vi "fucking PID.vi"(4 "lorentzian":T1={"Amplitude"=0.011556077084443558, "omega(0)"=1994480.3546612726, "Gamma"=468.65303298958196, "phase"=4.673413347310273, "Q"=4255.771784806969, "Norm  Ampl"=nan, "z (inf)"=2.6527949823343002e-05+0.0007477540585896028i, "4corners"={"z (-pi/2)"=9.277908004825974e-07+0.0007240755403629966i, "z(inf)"=2.6527949823343002e-05+0.0007477540585896028i, "z (pi/2)"=2.8494315967368497e-06+0.0007733542176124632i, "z center"=1.8886111986097237e-06+0.0007487148789877299i, "z(0)"=-2.2750727426123552e-05+0.000749675699385857i, "radius"=2.4658065287076567e-05}} {"z (inf)" format="%#9_9f"; "Q" format="%#9_9f"; "phase" format="%#9_9f"; "Gamma" format="%#9_9f"; "omega(0)" format="%#9_9f"}, 6 "requested size":i32=100, 7 "PID action":T3, 8 "voltage in (V)":cdb=-1.0+0.0i format="%#_10f", 9 "PID parameters":T4={"P (sec)"=-1.0, "I (sec)"=-1.0}, 10 "time in (sec)":dbl=-1.0, 11 "frequency in (Hz)":dbl=-1.0 format="%#_10f") -> (3 "frequency out (Hz)":dbl format="%#_10f")   [LabVIEW 2016]
uses:
  pid -- parameters.ctl
  agregator -- action.ctl
  lorentzian.ctl
  circle corners.ctl
  four-corner circle transformation.ctl
  Q -- check range -- i -- real.vi
  linear interpolation - real.vi
  Q - not nan -- real.vi
panel:
  out "delta theta":dbl
  out "actual number of elements":i32
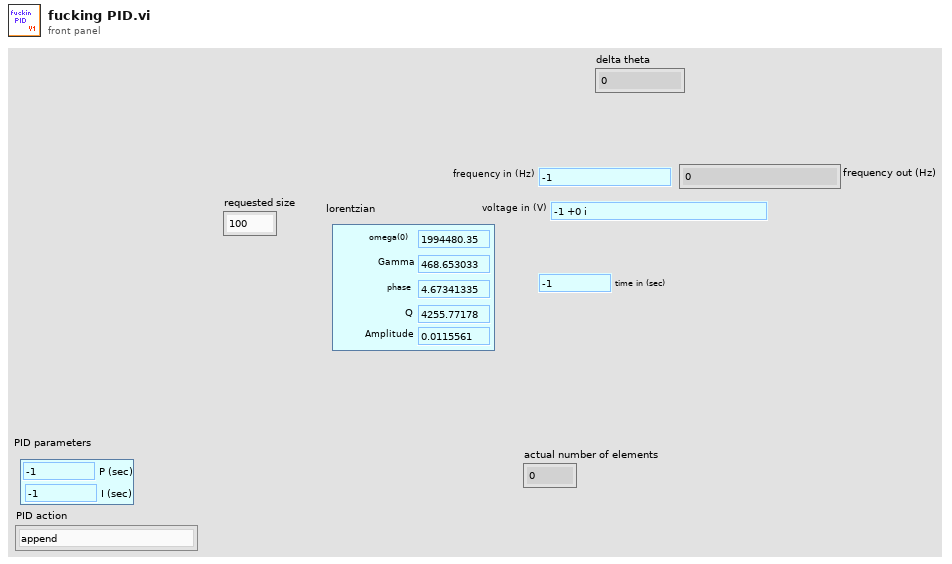
[diagram p1: front panel]
types:
  T1 = typedef "lorentzian.ctl" = cluster{"Amplitude":dbl, "omega(0)":dbl, "Gamma":dbl, "phase":dbl, "Q":dbl, "Norm  Ampl":dbl, "z (inf)":cdb, "4corners":T2}
  T2 = typedef "circle corners.ctl" = cluster{"z (-pi/2)":cdb, "z(inf)":cdb, "z (pi/2)":cdb, "z center":cdb, "z(0)":cdb, "radius":dbl}
  T3 = typedef "agregator -- action.ctl" = enum16{"append", "interpolate", "empty!", "force", "init", "scale", "read last"}
  T4 = typedef "pid -- parameters.ctl" = cluster{"P (sec)":dbl, "I (sec)":dbl}
  T5 = typedef "four-corner circle transformation.ctl" = enum16{"z(c) z(inf)", "z(c) z(zero)", "fix phase", "calculate lorentzian", "z(0) z(+-pi/2)", "shift to zcenter", "to  canonical", "get canonical phase"}
  T6 = typedef "interpolation state - real.ctl" = cluster{"requested size":i32, "Array":dbl[], "actual number of elements":i32}
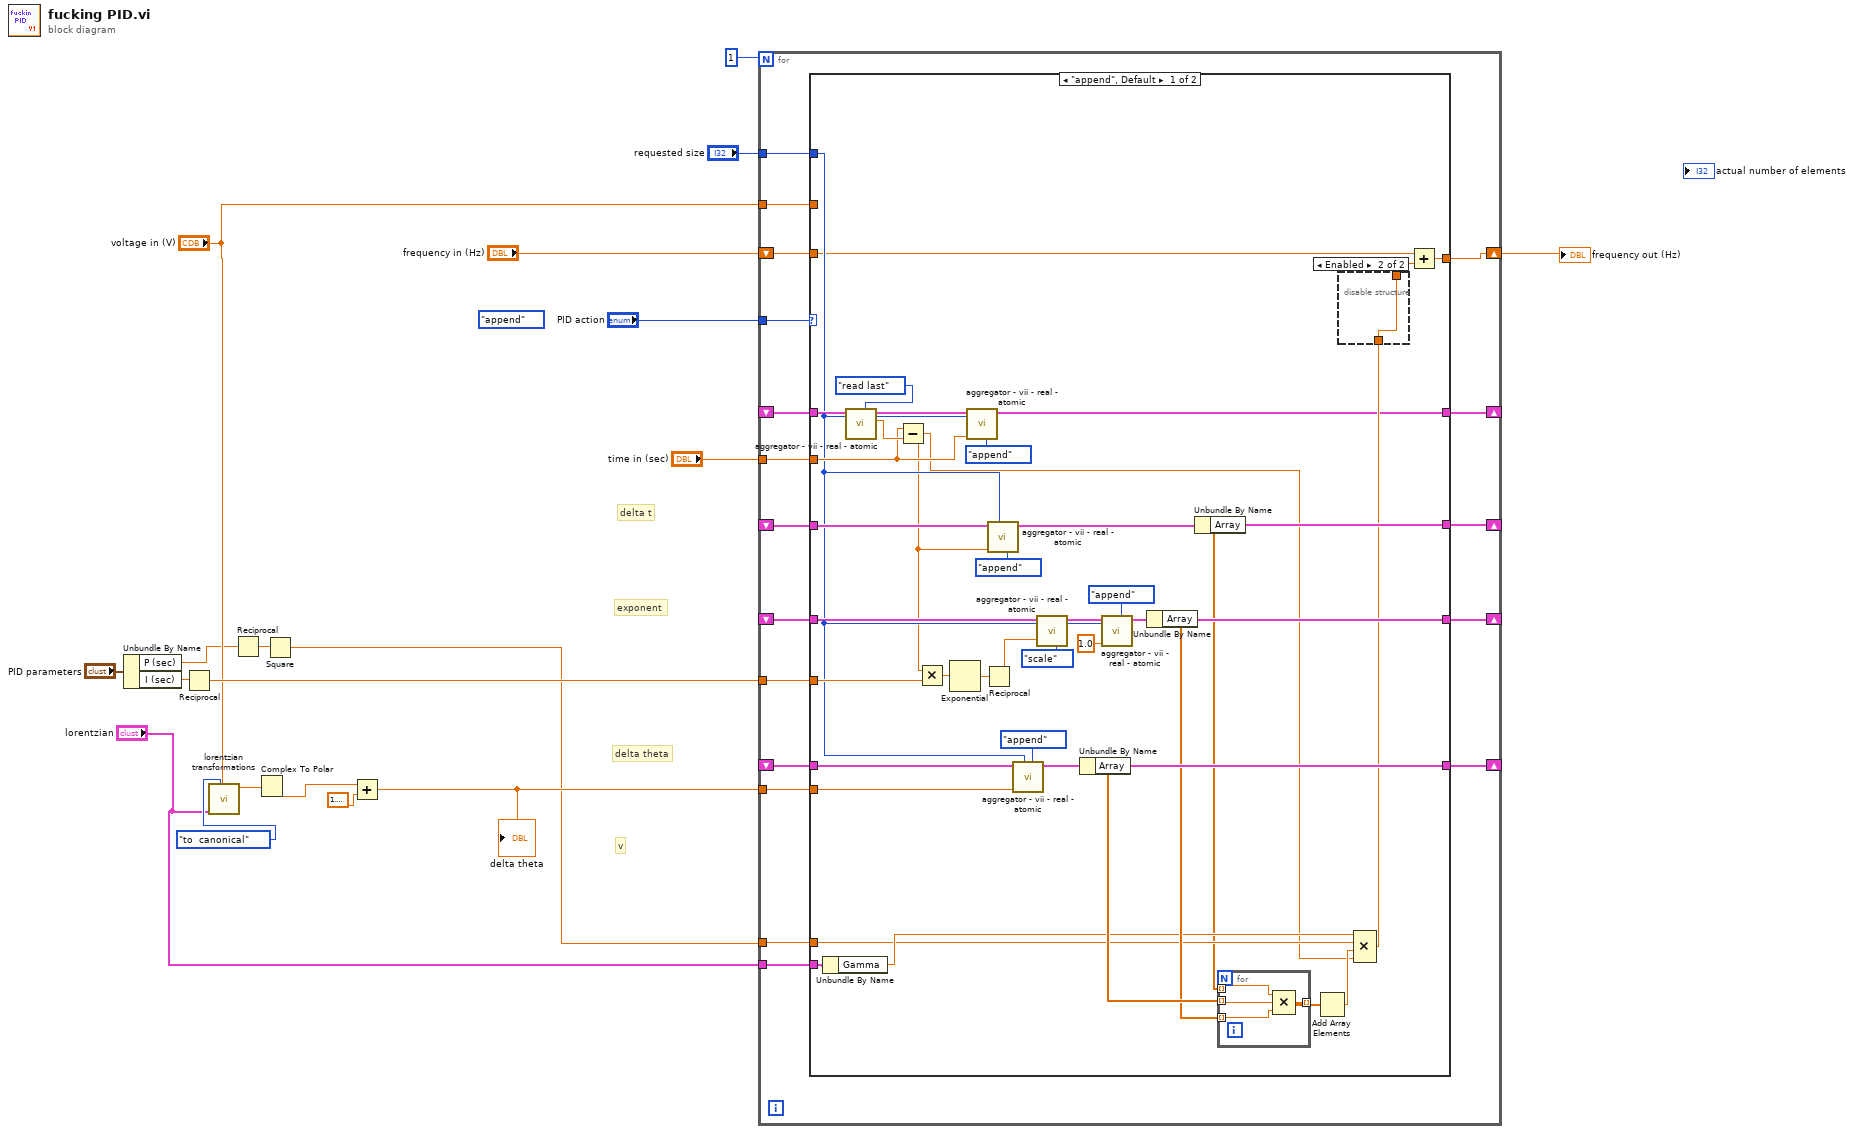
[diagram p0: block diagram]
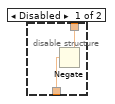
[diagram p2: hidden frame]
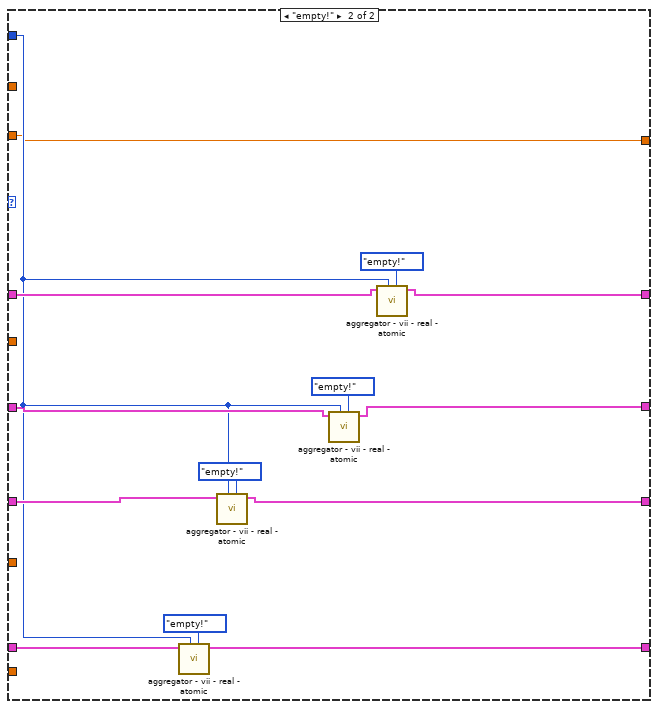
[diagram p3: hidden frame]
diagram:
  (unwired) agregator_--_action."append" ("aggregator action")
  # "v"
  # "delta theta"
  # "delta t"
  # "exponent"
  n1 = Unbundle By Name("PID parameters") -> ("P (sec)"=w4:dbl, "I (sec)"=w14:dbl)
  n2 = Reciprocal(x=w14) -> (1/x=w13:dbl)
  n3 = call "lorentzian transformations.vi"("4 corner circle transformation"=four-corner_circle_transformation."to  canonical", "lorentzian in"="lorentzian", "voltage in"="voltage in (V)") -> ("voltage out"=w9:cdb)  [unwired: 7 in, 1 out]
  n4 = Reciprocal(x=w4) -> (1/x=w3:dbl)
  n5 = Complex To Polar(r * e^(i*theta)=w9) -> (theta=w10:dbl)  [unwired: 1 out]
  n6 = Square(x=w3) -> (x^2=w2:dbl)
  n7 = Add(x=w10, y=1.5707963267948966) -> (x+y=w7:dbl)
  "delta theta" <- w7
  n8 = for {
    N: 1 -> [_]
    tunnel: "requested size" -> [w37]
    tunnel: "PID action" -> [w36]
    shift-right: [w34] -> _
    shift-left: _ -> [w35]
    tunnel: "time in (sec)" -> [w33]
    shift-right: [w31] -> _
    shift-left: _ -> [w32]
    tunnel: w13 -> [w30]
    tunnel: "voltage in (V)" -> [w29]
    shift-right: [w27] -> _
    shift-left: _ -> [w28]
    shift-right: [w24] -> _
    shift-left: _ -> [w26]
    tunnel: w7 -> [w25]
    tunnel: "lorentzian" -> [w22]
    tunnel: w2 -> [w21]
    shift-right: [w20] -> w1
    shift-left: "frequency in (Hz)" -> [w23]
    n9 = case shown="\"append\", Default" w36 {
      tunnel: w37 -> [w58 w84]
      tunnel: w35 -> [w75 w86]
      tunnel: [w38 w85] -> w34
      tunnel: w33 -> [w66 _]
      tunnel: w32 -> [w74 w90]
      tunnel: [w54 w89] -> w31
      tunnel: w30 -> [w65 _]
      tunnel: w29 -> [_ _]
      tunnel: w28 -> [w63 w88]
      tunnel: [w57 w87] -> w27
      tunnel: w26 -> [w62 w92]
      tunnel: w25 -> [w60 _]
      tunnel: [w59 w91] -> w24
      tunnel: w23 -> [w48 w83]
      tunnel: w22 -> [w52 _]
      tunnel: w21 -> [w50 _]
      tunnel: [w47 w83] -> w20
      frame "append", Default {
        n10 = Unbundle By Name(w52) -> ("Gamma"=w51:dbl)
        n11 = call "aggregator - vii - real - atomic.vi"("aggregator action"=agregator_--_action."read last", "requested size"=w58, "state IN"=w75) -> ("mean"=w68:dbl, "state OUT"=w46:T6)  [unwired: 5 in, 2 out]
        n12 = Subtract(x=w66, y=w68) -> (x-y=w41:dbl)
        n13 = Multiply(x=w41, y=w65) -> (x*y=w40:dbl)
        n14 = Exponential(1:w40) -> (0:w39:dbl)
        n15 = call "aggregator - vii - real - atomic.vi"("aggregator action"=agregator_--_action."append", "requested size"=w58, "number"=w66, "state IN"=w46) -> ("state OUT"=w38:T6)  [unwired: 4 in, 3 out]
        n16 = Reciprocal(x=w39) -> (1/x=w43:dbl)
        n17 = call "aggregator - vii - real - atomic.vi"("aggregator action"=agregator_--_action."append", "requested size"=w58, "number"=w41, "state IN"=w63) -> ("state OUT"=w57:T6)  [unwired: 4 in, 3 out]
        n18 = call "aggregator - vii - real - atomic.vi"("aggregator action"=agregator_--_action."append", "requested size"=w58, "number"=w60, "state IN"=w62) -> ("state OUT"=w59:T6)  [unwired: 4 in, 3 out]
        n19 = call "aggregator - vii - real - atomic.vi"("aggregator action"=agregator_--_action."scale", "requested size"=w58, "number"=w43, "state IN"=w74) -> ("state OUT"=w73:T6)  [unwired: 4 in, 3 out]
        n20 = Unbundle By Name(w59) -> ("Array"=w56:dbl[])
        n21 = call "aggregator - vii - real - atomic.vi"("aggregator action"=agregator_--_action."append", "requested size"=w58, "number"=1.0, "state IN"=w73) -> ("state OUT"=w54:T6)  [unwired: 4 in, 3 out]
        n22 = Unbundle By Name(w54) -> ("Array"=w53:dbl[])
        n23 = Unbundle By Name(w57) -> ("Array"=w42:dbl[])
        n24 = for {
          tunnel: w56 -> [w82] mode=indexing
          tunnel: [w81] -> w55 mode=indexing
          tunnel: w53 -> [w80] mode=indexing
          tunnel: w42 -> [w79] mode=indexing
          n25 = Compound Arithmetic op=MULTIPLY(w79, w82, w80) -> (w81:dbl)
        }
        n26 = Add Array Elements(numeric array=w55) -> (sum=w49:dbl)
        n27 = Compound Arithmetic op=MULTIPLY(w51, w50, w49, w41) -> (w45:dbl)
        n28 = disable-structure shown="Enabled" {
          disable-tunnel: w45 -> [w77 w78]
          disable-tunnel: [w76 w78] -> w44
          frame Disabled {
            n29 = Negate(x=w77) -> (-x=w76:dbl)
          }
          frame Enabled {
          }
        }
        n30 = Add(x=w48, y=w44) -> (x+y=w47:dbl)
      }
      frame "empty!" {
        n31 = call "aggregator - vii - real - atomic.vi"("aggregator action"=agregator_--_action."empty!", "requested size"=w84, "state IN"=w92) -> ("state OUT"=w91:T6)  [unwired: 5 in, 3 out]
        n32 = call "aggregator - vii - real - atomic.vi"("aggregator action"=agregator_--_action."empty!", "requested size"=w84, "state IN"=w90) -> ("state OUT"=w89:T6)  [unwired: 5 in, 3 out]
        n33 = call "aggregator - vii - real - atomic.vi"("aggregator action"=agregator_--_action."empty!", "requested size"=w84, "state IN"=w88) -> ("state OUT"=w87:T6)  [unwired: 5 in, 3 out]
        n34 = call "aggregator - vii - real - atomic.vi"("aggregator action"=agregator_--_action."empty!", "requested size"=w84, "state IN"=w86) -> ("state OUT"=w85:T6)  [unwired: 5 in, 3 out]
      }
    }
  }
  "frequency out (Hz)" <- w1
